vi "Write Param.vi"(8 "error in (no error)":errorcluster, 10 "Param":refnum<class "MB Param.lvclass">, 11 "MB_TCP in":refnum<class "Modbus Master CR.lvclass">) -> (0 "error out":errorcluster, 3 "MB_TCP out":refnum<class "Modbus Master CR.lvclass">)   [LabVIEW 2021, in "Modbus Master CR.lvclass"]
uses:
  Modbus Master CR.lvclass
  MB Param/MB Param/MB Param.lvclass
  Modbus Master CR.lvclass/Modbus Master CR.ctl
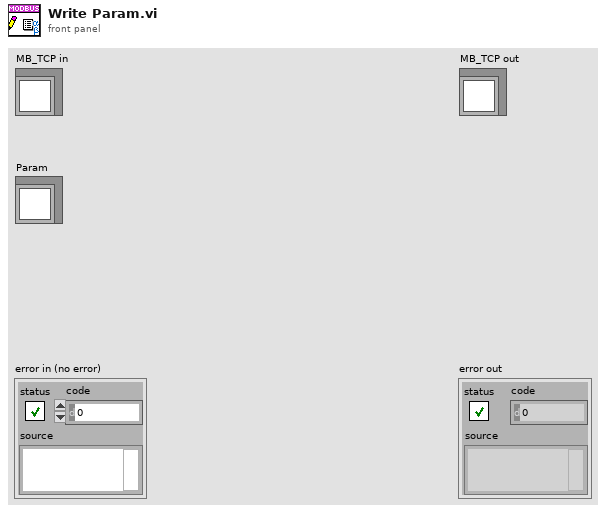
[diagram p1: front panel]
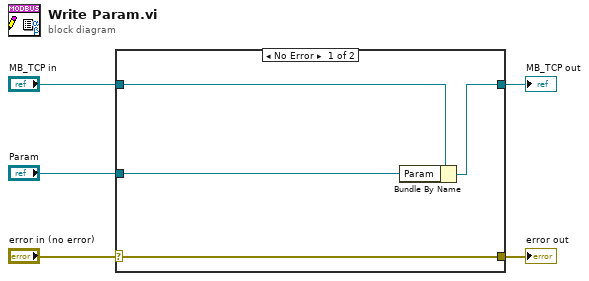
[diagram p0: block diagram]
diagram:
  n1 = case shown="No Error" "error in (no error)" {
    selector: "error in (no error)" -> [w9 w10]
    tunnel: [w9 w10] -> w4
    tunnel: [w7 w11] -> w2
    tunnel: "MB_TCP in" -> [w8 w11]
    tunnel: "Param" -> [w6 _]
    frame No Error {
      n2 = Bundle By Name(cluster=w8, "Param"=w6) -> (w7:refnum<class "Modbus Master CR.lvclass">)
    }
    frame Error {
    }
  }
  "error out" <- w4
  "MB_TCP out" <- w2
